vi "PH_BL-Master.PC _Boolean_Status_Subscriber_Status.vi"(0 "i ref in":refnum<vi>, 2 "Boolean Subscriber Instance Name":string="N/A", 3 "Status":T1 items=["no info", "off/false/out", "on/true/in", "Failure", "Alarm", "Status 1", "Status 2", "Status 3"], 4 "no Link?":bool, 5 "error in (no error)":errorcluster) -> (14 "i ref out":refnum<vi>, 19 "error out":errorcluster)   [LabVIEW 2014, in "PH_BL-Master.lvlib"]
doc: "This VI writes the incoming information aboutthe status of a status subscriber to own attributes."
uses:
  PH_BL-Master.lvlib
  PH_Basics/PH_StatusHandler/PH_StatusHandler.Status.ctl
  PH_Basics/PH_StatusHandler/PH_StatusHandler.lvlib
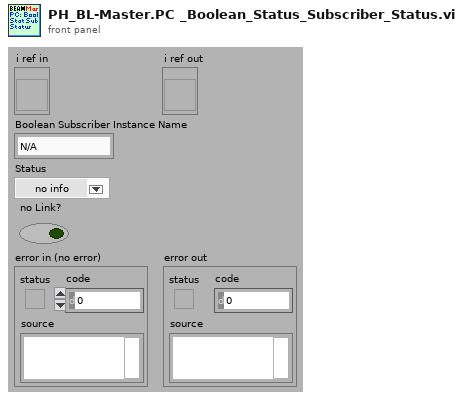
[diagram p1: front panel]
types:
  T1 = typedef "PH_StatusHandler.lvlib/PH_StatusHandler.Status.ctl" = i16
  T2 = typedef "PH_BL-Master.lvlib/PH_BL-Master.i attribute.ctl" = cluster{"Remote controlled":bool, "Boolean Condition Service Subscriber":refnum<vi>[], "Picture Condition Service Subscriber":refnum<vi>[], "R2S":cluster{"GUI Ref":refnum<vi>, "State":bool}, "Vacua":cluster{"GUI Ref":refnum<vi>, "Limit":dbl, "Curr Value":dbl, "in range":bool}[], "O2 Inspection":cluster{"GUI Ref":refnum<vi>, "Concentration":dbl, "State":T1}[], "Boolean Status Service Subscriber":cluster{"GUI Ref":refnum<vi>, "Status":T1, "no Link?":bool, "Status Subscriber Class":T3}[], "Picture Status Service Subscriber":cluster{"GUI Ref":refnum<vi>, "Status":T1, "no Link?":bool, "Status Subscriber Class":T3}[], "6P 4Q Service Subscriber":cluster{"GUI Ref":refnum<vi>, "Selector":T4, "no Link?":bool}[], "Index of latest 6P 4Q changing Instance":i32, "Index of latest Picture Status changing Instance":i32, "Index of latest Boolean Status changing Instance":i32, "Vision ID on same Node":string, "Start Phase over?":bool, "GUI Ref Delete":refnum<vi>}
  T3 = typedef "PH_BL-Master.lvlib/PH_BL-Master.Status Subscriber Class.ctl" = enum16{"unknown", "Switch", "BB", "6P Switch", "Switch GUI", "Switch and 6P State", "Force Sensor"}
  T4 = typedef "PH_4_Pos_Selector.lvlib/PH_4_Pos_Selector.Position Selector.ctl" = u16
  T5 = cluster{"GUI Ref":refnum<vi>, "Status":T1, "no Link?":bool, "Status Subscriber Class":T3}[]
  T6 = cluster{"GUI Ref":refnum<vi>, "Status":T1, "no Link?":bool, "Status Subscriber Class":T3}
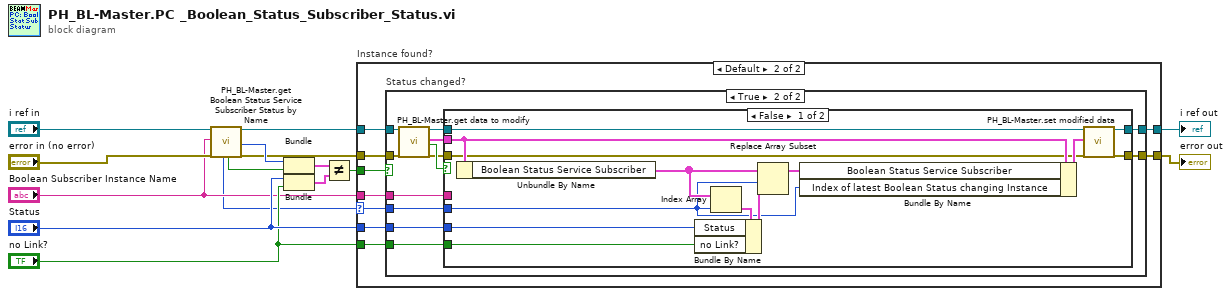
[diagram p0: block diagram]
diagram:
  n1 = call "PH_BL-Master.get Boolean Status Service Subscriber Status by Name.vi"("i ref in"="i ref in", "Status Subscriber Instance"="Boolean Subscriber Instance Name", "error in (no error)"="error in (no error)") -> ("index of element"=w1:i32, "no Link?"=w7:bool, "i ref out"=w5:refnum<vi>, "Subscriber State"=w8:T1, "error out"=w3:errorcluster)  [unwired: 7 in, 5 out]
  n2 = Bundle("Subscriber State"=w8, "no Link?"=w7) -> (w11:cluster{"Subscriber State":T1, "no Link?":bool})  [unwired: 1 in]
  n3 = Bundle("Status"="Status", "no Link?"="no Link?") -> (w12:cluster{"Status":T1, "no Link?":bool})  [unwired: 1 in]
  n4 = Not Equal?(x=w11, y=w12) -> (x != y?=w13:bool)
  n5 = case "Instance found?" shown="Default" w1 {
    selector: w1 -> [_ w21]
    tunnel: "Status" -> [_ w19]
    tunnel: [w16 w26] -> w15
    tunnel: [w17 w25] -> w14
    tunnel: w3 -> [w16 w24]
    tunnel: w5 -> [w17 w23]
    tunnel: "Boolean Subscriber Instance Name" -> [_ w22]
    tunnel: w13 -> [_ w20]
    tunnel: "no Link?" -> [_ w18]
    frame -1 {
    }
    frame Default {
      n6 = case "Status changed?" shown="True" w20 {
        tunnel: [w27 w36] -> w26
        tunnel: [w28 w35] -> w25
        tunnel: w24 -> [w27 w34]
        tunnel: w23 -> [w28 w33]
        tunnel: w22 -> [_ w32]
        tunnel: w21 -> [_ w31]
        tunnel: w19 -> [_ w30]
        tunnel: w18 -> [_ w29]
        frame False {
        }
        frame True {
          n7 = call "PH_BL-Master.get data to modify.vi"("i ref in"=w33, "error in (no error)"=w34) -> ("i ref out"=w37:refnum<vi>, "i attribute"=w39:T2, "timed out"=w40:bool, "error out"=w38:errorcluster)  [unwired: 14 in]
          n8 = case shown="False" w40 {
            tunnel: w37 -> [w41 w55]
            tunnel: [w53 w55] -> w35
            tunnel: w38 -> [w42 w54]
            tunnel: [w52 w54] -> w36
            tunnel: w39 -> [w51 _]
            tunnel: w30 -> [w49 _]
            tunnel: w31 -> [w43 _]
            tunnel: w32 -> [_ _]
            tunnel: w29 -> [w47 _]
            frame False {
              n9 = Unbundle By Name(w51) -> ("Boolean Status Service Subscriber"=w48:T5)
              n10 = Index Array(array=w48, index=w43) -> (element=w44:T6)
              n11 = Bundle By Name(cluster=w44, "Status"=w49, "no Link?"=w47) -> (w45:T6)
              n12 = Replace Array Subset(array=w48, new element=w45, index=w43) -> (w46:T5)
              n13 = Bundle By Name(cluster=w51, "Boolean Status Service Subscriber"=w46, "Index of latest Boolean Status changing Instance"=w43) -> (w50:T2)
              n14 = call "PH_BL-Master.set modified data.vi"("i ref in"=w41, "i attribute"=w50, "error in (no error)"=w42) -> ("i ref out"=w53:refnum<vi>, "error out"=w52:errorcluster)  [unwired: 15 in]
            }
            frame True {
            }
          }
        }
      }
    }
  }
  "error out" <- w15
  "i ref out" <- w14
